vi "Contour Line Plot.vi"() -> ()   [LabVIEW 2023]
doc: "Demonstrates the use of the Contour Line VI to draw contours of multiple sample models, including a circle, sin(x)*sin*(y), and a 2D Peak function."
uses:
  <vilib>/Analysis/1siggen.llb/Ramp Pattern by Samples.vi
  <vilib>/Analysis/geometry.llb/Contour Line (Number of Heights).vi
  <vilib>/Analysis/NI_AAL_Geometry.lvlib
  <vilib>/Analysis/NI_AALBase.lvlib
panel:
  out "Contour Line":cluster{dbl[], dbl[]}[](graph)
  out "Surface":dbl[][](graph)
  in  "# of heights":i32=9 min=1 max=1000
  in  "surface model":u16(ring)=2 items=["Circle", "Sin X * Sin Y", "2D Peak Function"]
  # "Overview: Demonstrates the use of the Contour Line VI.\nRequirements: LabVIEW Full Development System\nInstructions: \n1. Use the surface model options to choose the surface and contour lines to display. \n2. Change # of heights to set the number of height levels in the Contour Line graph.\n3. Run the VI."
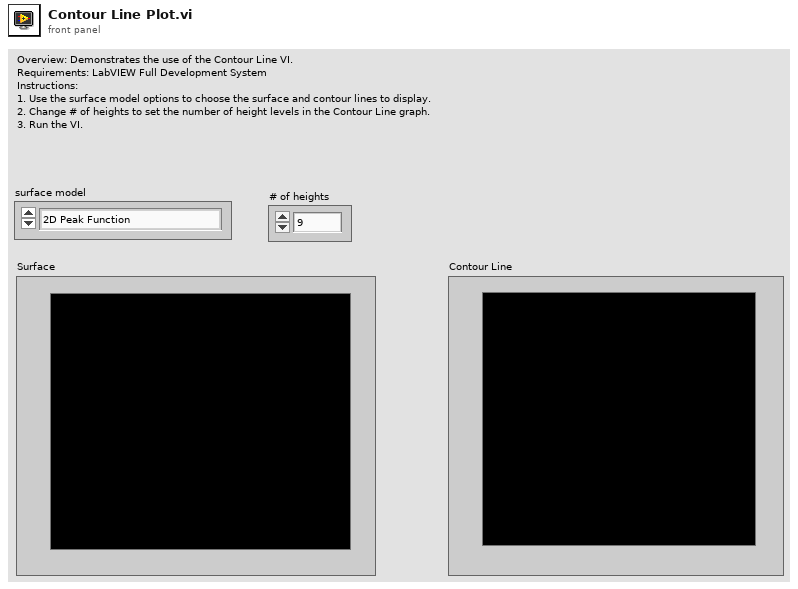
[diagram p1: front panel]
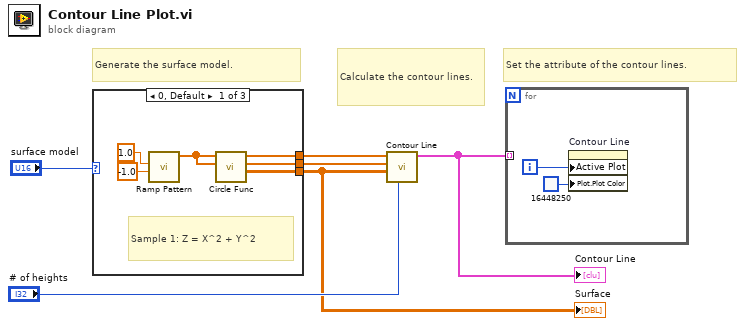
[diagram p0: block diagram]
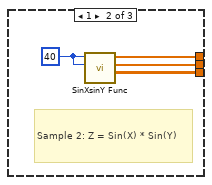
[diagram p2: hidden frame]
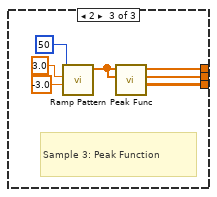
[diagram p3: hidden frame]
diagram:
  # "Generate the surface model."
  # "Calculate the contour lines."
  # "Set the attribute of the contour lines."
  n1 = case shown="0, Default" "surface model" {
    tunnel: [w9 w15 w19] -> w5
    tunnel: [w8 w14 w18] -> w4
    tunnel: [w7 w13 w17] -> w1
    frame 0, Default {
      # "Sample 1: Z = X^2 + Y^2"
      n2 = call-poly <vilib>:"Ramp Pattern.vi"("start"=-1.0, "end"=1.0) -> ("Ramp Pattern"=w10:dbl[])  [unwired: 8 in, 1 out]
      n3 = call "Circle Func.vi"("Y In"=w10, "X In"=w10) -> ("Z"=w7:dbl[][], "Y Out"=w8:dbl[], "X Out"=w9:dbl[])  [unwired: 7 in]
    }
    frame 1 {
      w16 = 40 ("X length")
      # "Sample 2: Z = Sin(X) * Sin(Y)"
      n4 = call "SinXsinY Func.vi"("Y length"=w16, "X length"=w16) -> ("Z"=w13:dbl[][], "Y Out"=w14:dbl[], "X Out"=w15:dbl[])  [unwired: 7 in]
    }
    frame 2 {
      # "Sample 3: Peak Function"
      n5 = call-poly <vilib>:"Ramp Pattern.vi"("start"=-3.0, "end"=3.0, "samples"=50) -> ("Ramp Pattern"=w21:dbl[])  [unwired: 7 in, 1 out]
      n6 = call "Peak Func.vi"("Y In"=w21, "X In"=w21) -> ("Z"=w17:dbl[][], "Y Out"=w18:dbl[], "X Out"=w19:dbl[])  [unwired: 7 in]
    }
  }
  "Surface" <- w1
  n7 = call-poly <vilib>:"Contour Line.vi"("number of heights"="# of heights", "Z"=w1, "Y"=w4, "X"=w5) -> ("Contour Graph"=w2:cluster{dbl[], dbl[]}[])  [unwired: 5 in, 2 out]
  "Contour Line" <- w2
  n8 = for {
    tunnel: w2 -> [_] mode=indexing
    i -> [w25]
    n9 = property on="Contour Line" class="XYGraph (strict)"("Active Plot"=w25, "Plot.Plot Color"=u32 16448250) -> ()  [unwired: 2 in, 2 out]
  }
